vi "multi-graph-plot.vi"() -> ()   [LabVIEW 2025]
uses:
  <vilib>/numeric/Random Number (Range) U64.vi
  <vilib>/numeric/sub_Random U32.vi
panel:
  out "Waveform Chart":T1(graph)
  in  "stop":bool
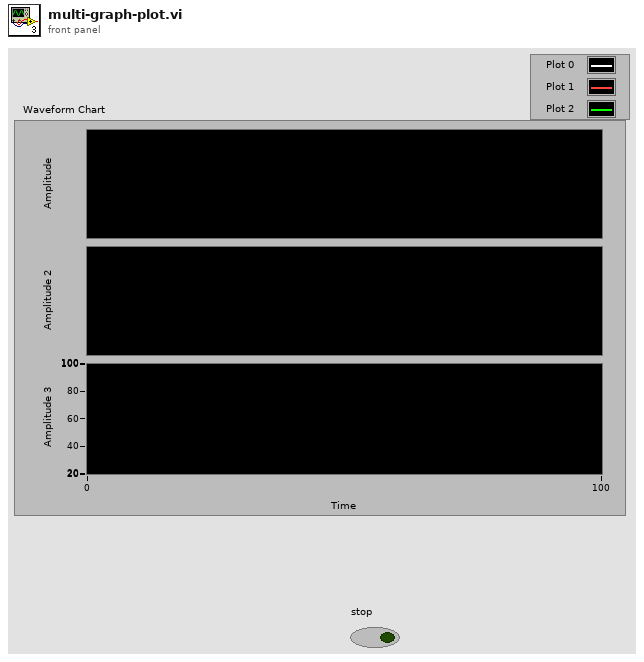
[diagram p1: front panel]
types:
  T1 = cluster{"number":u64, "number":u64, "number":u64}
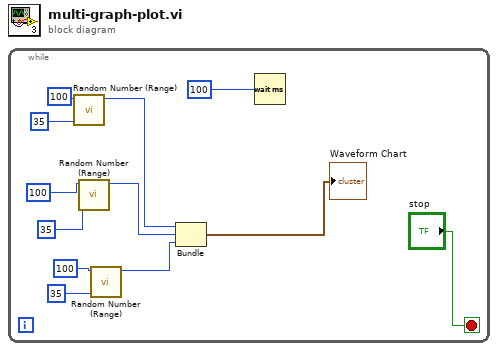
[diagram p0: block diagram]
diagram:
  n1 = while {
    stop <- "stop" stop-if-true
    n2 = call-poly <vilib>:"Random Number (Range).vi"("lower bound (0)"=u64 35, "upper bound (100)"=u64 100) -> ("number"=w6:u64)  [unwired: 9 in]
    n3 = call-poly <vilib>:"Random Number (Range).vi"("lower bound (0)"=u64 35, "upper bound (100)"=u64 100) -> ("number"=w5:u64)  [unwired: 9 in]
    n4 = call-poly <vilib>:"Random Number (Range).vi"("lower bound (0)"=u64 35, "upper bound (100)"=u64 100) -> ("number"=w4:u64)  [unwired: 9 in]
    n5 = Bundle("number"=w6, "number"=w5, "number"=w4) -> (→"Waveform Chart":T1)  [unwired: 1 in]
    n6 = Wait (ms)(milliseconds to wait=u32 100 ("millisecond timer value")) -> ()  [unwired: 1 out]
  }
